vi "Run Core.vi"(8 "Error In":errorcluster, 9 "Timeout (s)":dbl, 10 "Meas In":refnum<class "AbstractLogMessage.lvclass">, 11 "Hardware In":refnum<class "ILogger.lvclass">) -> (0 "Error Out":errorcluster, 1 "Timeout?":bool, 2 "Result Out":refnum<class "IResult.lvclass">, 3 "Hardware Out":refnum<class "ILogger.lvclass">)   [LabVIEW 2020, in "AbstractLogMessage.lvclass"]
uses:
  IResult/IResult.lvclass
  AbstractLogMessage.lvclass
  ILogger/ILogger.lvclass
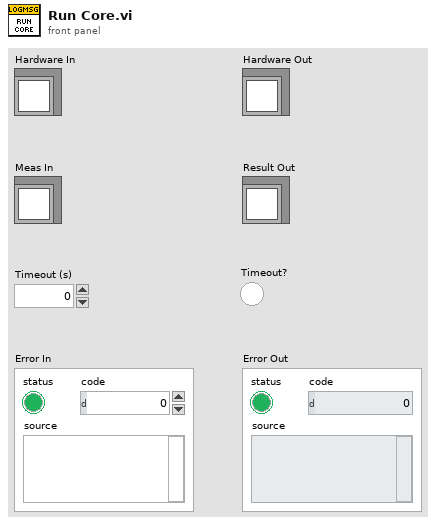
[diagram p1: front panel]
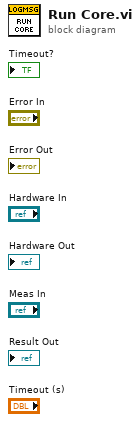
[diagram p0: block diagram]
diagram:
